vi "host_chat.vi"() -> (0 "cancel":bool, 1 "host":bool, 3 "username":string)   [LabVIEW 2024]
panel:
  in  "cancel":bool
  in  "send":bool
  in  "USERNAME":string
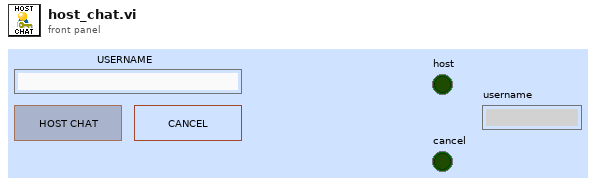
[diagram p1: front panel]
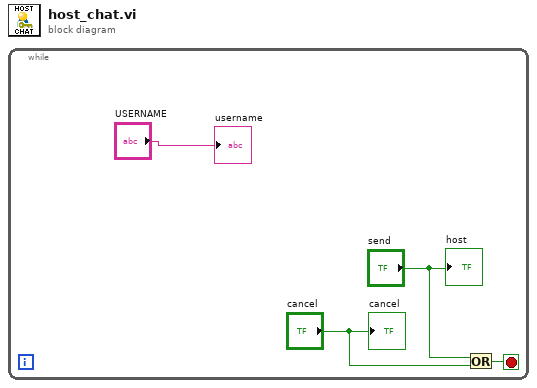
[diagram p0: block diagram]
diagram:
  n1 = while {
    stop <- w4 stop-if-true
    n2 = Or(x="send", y="cancel") -> (x .or. y?=w4:bool)
    "host" <- "send"
    "cancel" <- "cancel"
    "username" <- "USERNAME"
  }
